vi "Write VData.vi"(8 "error in (no error)":errorcluster, 10 "VData":variant, 11 "EnumeratedVariant in":refnum<class "EnumeratedVariant.lvclass">) -> (0 "error out":errorcluster, 3 "EnumeratedVariant out":refnum<class "EnumeratedVariant.lvclass">)   [LabVIEW 2020, in "EnumeratedVariant.lvclass"]
uses:
  EnumeratedVariant.lvclass
  EnumeratedVariant.lvclass/EnumeratedVariant.ctl
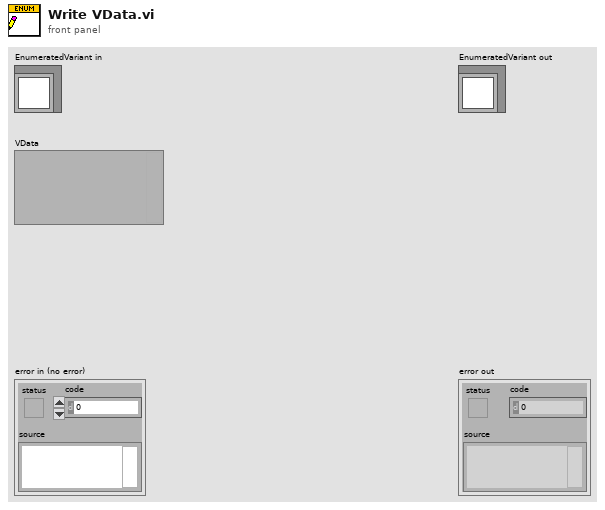
[diagram p1: front panel]
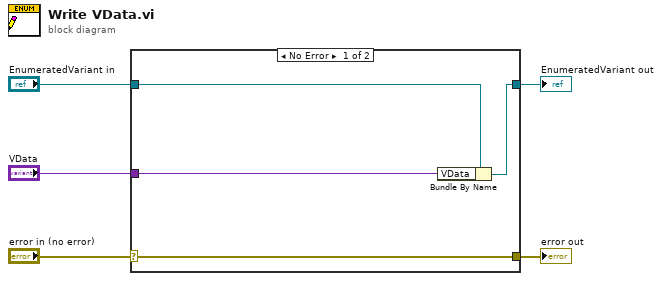
[diagram p0: block diagram]
diagram:
  n1 = case shown="No Error" "error in (no error)" {
    selector: "error in (no error)" -> [w9 w10]
    tunnel: [w9 w10] -> w4
    tunnel: [w7 w11] -> w2
    tunnel: "EnumeratedVariant in" -> [w8 w11]
    tunnel: "VData" -> [w6 _]
    frame No Error {
      n2 = Bundle By Name(cluster=w8, "VData"=w6) -> (w7:refnum<class "EnumeratedVariant.lvclass">)
    }
    frame Error {
    }
  }
  "error out" <- w4
  "EnumeratedVariant out" <- w2
